vi "programa 4.vi"() -> ()   [LabVIEW 2011]
panel:
  out "Rango":string
  out "121-180":bool
  out "81-120":bool
  out "1-80":bool
  out "Velocidad":dbl(knob) scale=0.0..180.0
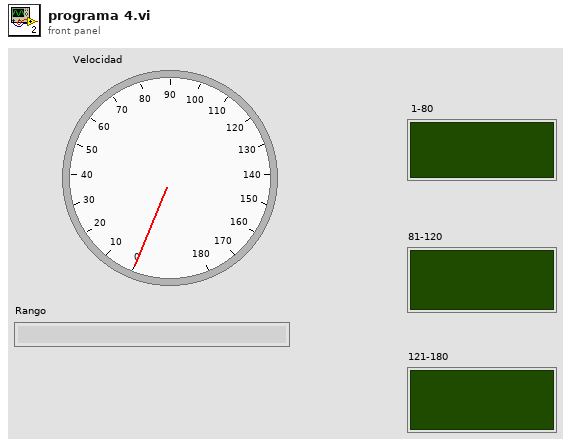
[diagram p1: front panel]
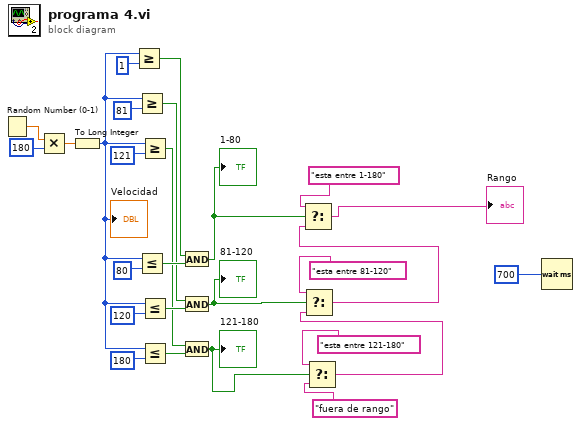
[diagram p0: block diagram]
diagram:
  n1 = Random Number (0-1)() -> (number: 0 to 1=w26:dbl)
  n2 = Multiply(x=w26, y=180) -> (x*y=w27:dbl)
  n3 = To Long Integer(number=w27) -> (32bit integer=w16:i32)
  "Velocidad" <- w16
  n4 = Greater Or Equal?(x=w16, y=1) -> (x >= y?=w22:bool)
  n5 = Greater Or Equal?(x=w16, y=81) -> (x >= y?=w19:bool)
  n6 = Less Or Equal?(x=w16, y=80) -> (x <= y?=w21:bool)
  n7 = Greater Or Equal?(x=w16, y=121) -> (x >= y?=w13:bool)
  n8 = Less Or Equal?(x=w16, y=120) -> (x <= y?=w20:bool)
  n9 = Less Or Equal?(x=w16, y=180) -> (x <= y?=w12:bool)
  n10 = And(x=w22, y=w21) -> (x .and. y?=w11:bool)
  "1-80" <- w11
  n11 = And(x=w19, y=w20) -> (x .and. y?=w6:bool)
  "81-120" <- w6
  n12 = And(x=w13, y=w12) -> (x .and. y?=w4:bool)
  "121-180" <- w4
  n13 = Select(t="esta entre 121-180", s=w4, f="fuera de rango") -> (s? t:f=w1:string)
  n14 = Select(t="esta entre 81-120", s=w6, f=w1) -> (s? t:f=w8:string)
  n15 = Select(t="esta entre 1-180", s=w11, f=w8) -> (s? t:f=→"Rango":string)
  n16 = Wait (ms)(milliseconds to wait=u32 700 ("millisecond timer value")) -> ()  [unwired: 1 out]
